vi "INTELLIFAUCET_Manipulate Variable to uA.vi"(10 "MV":dbl) -> (3 "4-20uA Output":i32)   [LabVIEW 2023]
uses:
  <vilib>/addons/control/pid/pid.llb/PID Percentage to EGU (DBL).vi
  <vilib>/addons/control/pid/NI_PID_pid.lvlib
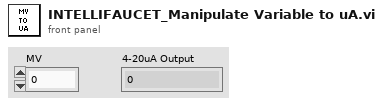
[diagram p1: front panel]
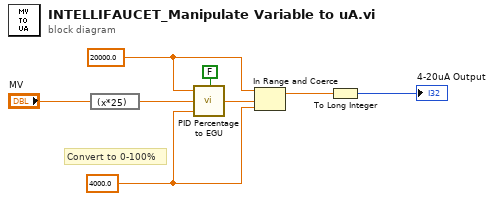
[diagram p0: block diagram]
diagram:
  w5 = 20000.0 ("Max")
  w4 = 4000.0 ("Min")
  # "Convert to 0-100%"
  n1 = expression code="(x*25)"("MV") -> (w6:dbl)
  n2 = call-poly <vilib>:"PID Percentage to EGU.vi"("coerce output to range? (T)"=FALSE, "minimum (EGU)"=w4, "% span"=w6, "maximum (EGU)"=w5) -> ("output (EGU)"=w3:dbl)
  n3 = In Range and Coerce(upper limit=w5, x=w3, lower limit=w4) -> (coerced(x)=w2:dbl)  [unwired: 1 out]
  n4 = To Long Integer(number=w2) -> (32bit integer=→"4-20uA Output":i32)
